vi "Steering Motor Encoder Read.vi"(6 "Configuration":T1={"Accelerometer Bias"={"X (m/s)"=0.0, "Y (m/s)"=0.0, "Z (m/s)"=0.0}, "Gyroscope Bias"={"X (m/s)"=0.0, "Y (m/s)"=0.0, "Z (m/s)"=0.0}, "Steering Motor Gear Ratio"=111.0, "Steering Pully Gear Ratio"=1.0, "Steering Encoder CPR"=500.0, "Steering Motor Max RPM"=4000.0, "Wheelbase (m)"=1.12, "Fork Angle (rad)"=1.3, "Balancing Controller"={"Kp (/s)"=0.0, "Kd (1)"=0.0}, "Max Allowed Steering Angle (rad)"=0.7, "Task Periods"={"Emergency Stop (us)"=0, "IMU (us)"=0, "Steering Motor Encoder (us)"=0, "State Estimator (us)"=0, "Balancing Controller (us)"=0, "GNSS (us)"=0, "Logging (us)"=0, "Drive Motor (us)"=0}, "Drive Motor Gear Ratio"=0.7, "Drive Motor UART Delay (ms)"=10, "Parameters"={"Numeric"=0.0}}, 8 "Measurement In":refnum<data-value>, 9 "Flag Steering Encoder":dbl, 10 "Reset Counter":bool, 11 "Error In":errorcluster) -> (0 "Measurement Out":refnum<data-value>, 1 "Steering Motor Encoder Data":T2, 3 "Error Out":errorcluster)   [LabVIEW 2021]
uses:
  <vilib>/myRIO/Common/Instrument Driver Framework/myRIO v1.0/Encoder/typedefs/Encoder Count Direction Enum.ctl
  <vilib>/myRIO/Common/Instrument Driver Framework/myRIO v1.0/Encoder/typedefs/Encoder Signal Mode.ctl
  <vilib>/myRIO/Common/Instrument Driver Framework/myRIO v1.0/Encoder/typedefs/Encoder Channels Enum.ctl
  <vilib>/myRIO/Common/Instrument Driver Framework/Utilities/typedefs/Generic FPGA Reference.ctl
  <vilib>/myRIO/Common/Instrument Driver Framework/Utilities/typedefs/myRIO v1.0 Reference.ctl
  <vilib>/myRIO/Common/Instrument Driver Framework/Utilities/typedefs/Hardware Version Enum.ctl
  <vilib>/myRIO/Common/Instrument Driver Framework/Utilities/typedefs/myRIO Generic Hardware Reference.ctl
  <vilib>/myRIO/Instrument Drivers/Onboard IO/Encoder/typedefs/Encoder Reference.ctl
  <vilib>/myRIO/Instrument Drivers/Onboard IO/Encoder/Encoder.lvlib
  <vilib>/myRIO/Instrument Drivers/Onboard IO/Encoder/vis/Read.vi
  <vilib>/myRIO/Instrument Drivers/Onboard IO/Encoder/vis/myRIO Encoder Open.xnode
  <vilib>/myRIO/Common/Instrument Driver Framework/Utilities/vis/Is FPGA Ref Available.vi
  <vilib>/myRIO/Express VI/Onboard IO/Encoder/Encoder Express VI.xnode
  Logging/Log Level.ctl
  <vilib>/myRIO/Common/Instrument Driver Framework/myRIO v1.0/Encoder/vis/myRIO v1.1 Open Encoder.vi
  <vilib>/myRIO/Common/Instrument Driver Framework/myRIO v1.0/Encoder/vis/myRIO v1.0 Configure Encoder.vi
  <vilib>/myRIO/Common/Instrument Driver Framework/myRIO v1.0/Encoder/typedefs/Encoder Configuration v1.0.ctl
  <vilib>/userDefined/High Color/nirio_resource_hc.ctl
  Steering Motor Encoder Data.ctl
  Configuration/Configuration.ctl
  GNSS/GNSS Data.ctl
  IMU/IMU Data.ctl
  State Estimator/Measurements.ctl
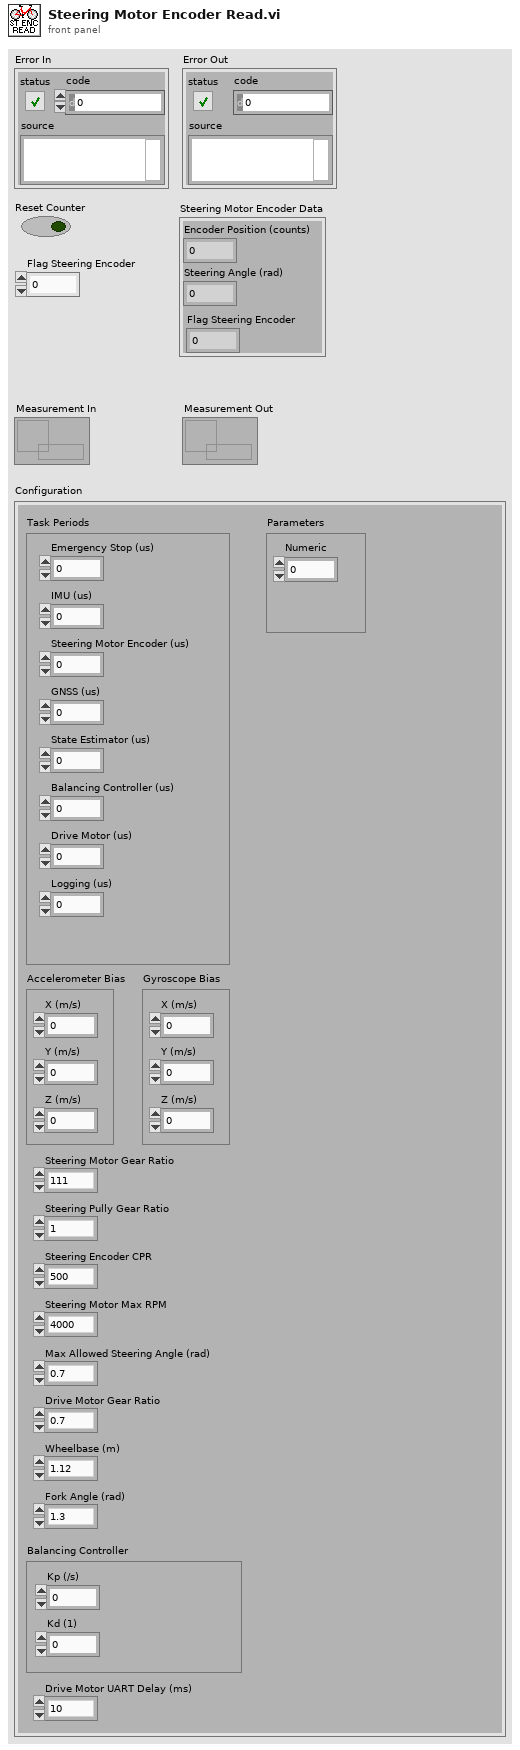
[diagram p1: front panel]
types:
  T1 = typedef "Configuration.ctl" = cluster{"Accelerometer Bias":cluster{"X (m/s)":dbl, "Y (m/s)":dbl, "Z (m/s)":dbl}, "Gyroscope Bias":cluster{"X (m/s)":dbl, "Y (m/s)":dbl, "Z (m/s)":dbl}, "Steering Motor Gear Ratio":dbl, "Steering Pully Gear Ratio":dbl, "Steering Encoder CPR":dbl, "Steering Motor Max RPM":dbl, "Wheelbase (m)":dbl, "Fork Angle (rad)":dbl, "Balancing Controller":cluster{"Kp (/s)":dbl, "Kd (1)":dbl}, "Max Allowed Steering Angle (rad)":dbl, "Task Periods":cluster{"Emergency Stop (us)":i64, "IMU (us)":i64, "Steering Motor Encoder (us)":i64, "State Estimator (us)":i64, "Balancing Controller (us)":i64, "GNSS (us)":i64, "Logging (us)":i64, "Drive Motor (us)":i64}, "Drive Motor Gear Ratio":dbl, "Drive Motor UART Delay (ms)":i64, "Parameters":cluster{"Numeric":dbl}}
  T2 = typedef "Steering Motor Encoder Data.ctl" = cluster{"Encoder Position (counts)":i32, "Steering Angle (rad)":dbl, "Flag Steering Encoder":dbl}
  T3 = typedef "Log Level.ctl" = enum16{"Error", "Warning", "Info"}
  T4 = typedef "Measurements.ctl" = cluster{"IMU Data":T5, "Steering Motor Encoder Data":T2, "GNSS Data":T6}
  T5 = typedef "IMU Data.ctl" = cluster{"Gyroscope":cluster{"X (rad/s)":dbl, "Y (rad/s)":dbl, "Z (rad/s)":dbl}, "Accelerometer":cluster{"X (m/s^2)":dbl, "Y (m/s^2)":dbl, "Z (m/s^2)":dbl}, "Flag IMU":dbl}
  T6 = typedef "GNSS Data.ctl" = cluster{"Latitude (rad)":dbl, "Longitude (rad)":dbl, "Altitude (m)":dbl, "Speed (m/s)":dbl, "Heading (rad)":dbl, "Fix Quality":i32, "Number of Satellites":i32, "Latitude (deg)":dbl, "Longitude (deg)":dbl, "Flag GNSS":dbl}
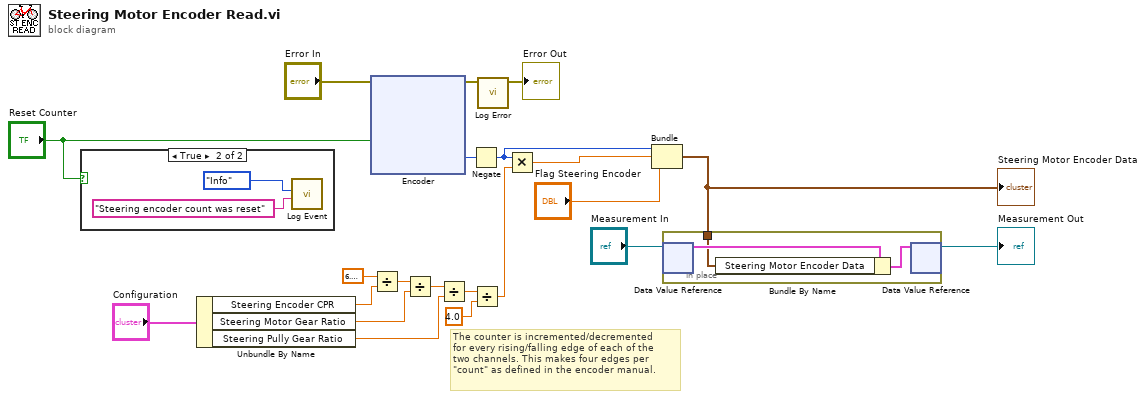
[diagram p0: block diagram]
diagram:
  # "The counter is incremented/decremented\nfor every rising/falling edge of each of the\ntwo channels. This makes four edges per\n\"count\" as defined in the encoder manual."
  n1 = case shown="True" "Reset Counter" {
    frame False {
    }
    frame True {
      n2 = call "Log Event.vi"("Message"="Steering encoder count was reset", "Log Level"=Log_Level."Info") -> ()  [unwired: 9 in, 1 out]
    }
  }
  n3 = Unbundle By Name("Configuration") -> ("Steering Encoder CPR"=w15:dbl, "Steering Motor Gear Ratio"=w13:dbl, "Steering Pully Gear Ratio"=w11:dbl)
  n4 = xnode "Encoder"("Reset Counter"="Reset Counter", "error in (no error)"="Error In") -> ("Counter Value"=w20:i32, "error out"=w4:errorcluster)  [unwired: 2 out]
  n5 = Divide(x=6.283185307179586, y=w15) -> (x/y=w14:dbl)
  n6 = Divide(x=w14, y=w13) -> (x/y=w12:dbl)
  n7 = Divide(x=w12, y=w11) -> (x/y=w10:dbl)
  n8 = Negate(x=w20) -> (-x=w18:i32)
  n9 = Divide(x=w10, y=4.0) -> (x/y=w9:dbl)
  n10 = call "Log Error.vi"("Error In"=w4) -> ("Error Out"=→"Error Out":errorcluster)  [unwired: 10 in]
  n11 = Multiply(x=w18, y=w9) -> (x*y=w19:dbl)
  n12 = Bundle(w18, w19, "Flag Steering Encoder"="Flag Steering Encoder") -> (w5:cluster{i32, dbl, "Flag Steering Encoder":dbl})  [unwired: 1 in]
  "Steering Motor Encoder Data" <- w5
  n13 = in-place {
    in-place-border: w5 -> [w24]
    n14 = in-place-dvr #1("Measurement In") -> (w26:T4)  [unwired: 1 out]
    n15 = Bundle By Name(cluster=w26, "Steering Motor Encoder Data"=w24) -> (w25:T4)
    n16 = in-place-dvr #1(w25) -> (→"Measurement Out":refnum<data-value>)  [unwired: 1 out]
  }
